vi "array keep.vi"(4 "slope win":dbl(slide)=90.0 scale=0.0..180.0, 6 "slope B":dbl(slide)=90.0 scale=0.0..180.0, 10 "Y":dbl[](array[numeric]), 11 "X":dbl[](array[numeric])) -> (2 "Y out":dbl[](array[numeric]), 3 "X out":dbl[](array[numeric]))   [LabVIEW 2020]
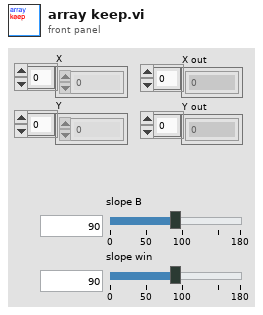
[diagram p1: front panel]
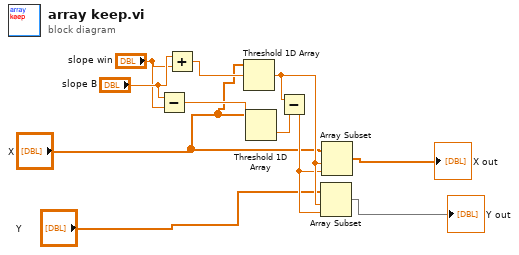
[diagram p0: block diagram]
diagram:
  n1 = Subtract(x="slope B", y="slope win") -> (x-y=w8:dbl)
  n2 = Add(x="slope B", y="slope win") -> (x+y=w9:dbl)
  n3 = Threshold 1D Array(2:w9, 3:"X") -> (0:w6:dbl)  [unwired: 1 in]
  n4 = Threshold 1D Array(2:w8, 3:"X") -> (0:w7:dbl)  [unwired: 1 in]
  n5 = Subtract(x=w6, y=w7) -> (x-y=w5:dbl)
  n6 = Array Subset(array="Y", index=w6, length=w5) -> (→"Y out":dbl[])
  n7 = Array Subset(array="X", index=w6, length=w5) -> (→"X out":dbl[])
